vi "Close Labels.vi"(8 "error in (no error)":errorcluster, 11 "Labels Reference In":T1) -> (0 "error out":errorcluster)   [LabVIEW 2018]
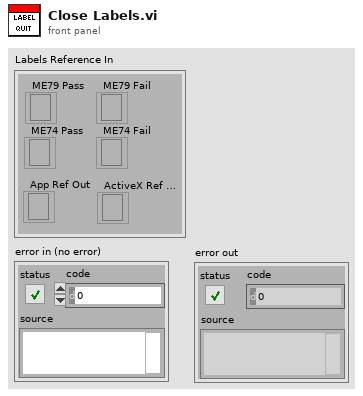
[diagram p1: front panel]
types:
  T1 = cluster{"ME79 Pass":refnum<k7>, "ME79 Fail":refnum<k7>, "ME74 Pass":refnum<k7>, "ME74 Fail":refnum<k7>, "App Ref Out":refnum<k7>, "ActiveX Ref Out":refnum<k7>}
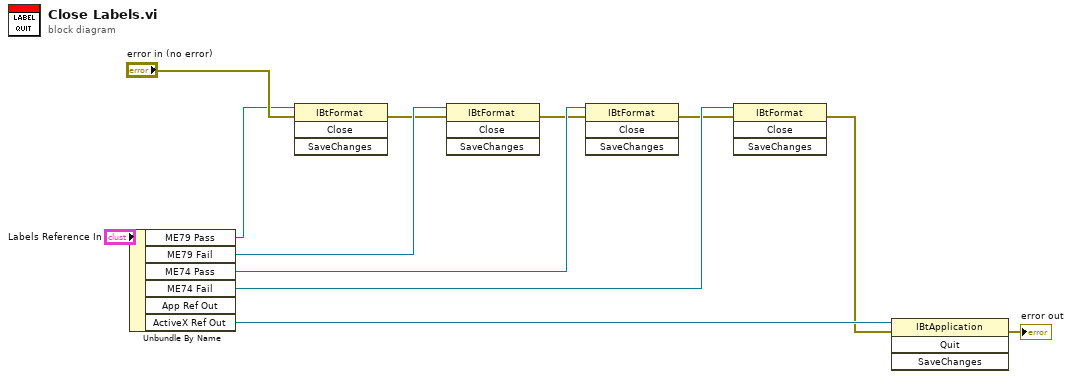
[diagram p0: block diagram]
diagram:
  n1 = Unbundle By Name("Labels Reference In") -> ("ME79 Pass"=w10:refnum<k7>, "ME79 Fail"=w9:refnum<k7>, "ME74 Pass"=w8:refnum<k7>, "ME74 Fail"=w7:refnum<k7>, "ActiveX Ref Out"=w3:refnum<k7>)  [unwired: 1 out]
  n2 = invoke class="IBtFormat" method="Close"(reference=w10, error in="error in (no error)") -> (error out=w6:errorcluster)  [unwired: 2 in, 3 out]
  n3 = invoke class="IBtFormat" method="Close"(reference=w9, error in=w6) -> (error out=w5:errorcluster)  [unwired: 2 in, 3 out]
  n4 = invoke class="IBtFormat" method="Close"(reference=w8, error in=w5) -> (error out=w4:errorcluster)  [unwired: 2 in, 3 out]
  n5 = invoke class="IBtFormat" method="Close"(reference=w7, error in=w4) -> (error out=w2:errorcluster)  [unwired: 2 in, 3 out]
  n6 = invoke class="IBtApplication" method="Quit"(reference=w3, error in=w2) -> (error out=→"error out":errorcluster)  [unwired: 2 in, 3 out]
